vi "N5700 Reset.vi"(5 "error":errorcluster, 8 "VISA":refnum<visa-resource-name>) -> (0 "error out":errorcluster, 3 "VISA out":refnum<visa-resource-name>)   [LabVIEW 2020]
doc: "This VI resets the N5700 power supply to a precise and safe state. \n\nThe reset state includes:\n- Output off\n- Voltage program limit to zero\n- Current program limit to zero\n- Over-voltage protection setting to maximum\n- Under-voltage limit to zero\n- Over-current protection off\n\nStatus registers are not reset"
panel:
  in  "Command":string="*RST"
  # "Agilent Technologies  \nSeries N5700A\n  DC Power Supplies"
  # "Reset Power Supply"
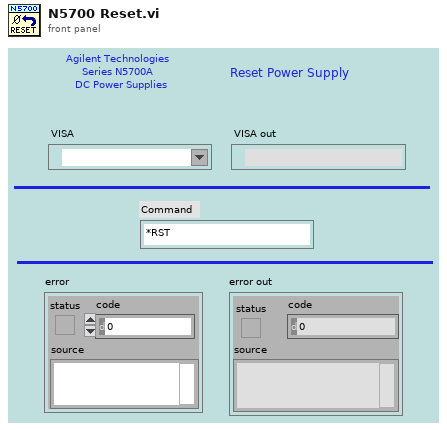
[diagram p1: front panel]
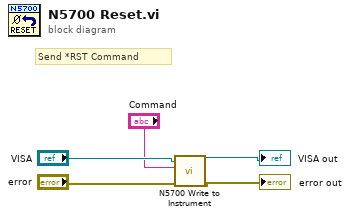
[diagram p0: block diagram]
diagram:
  # "Send *RST Command"
  n1 = call "N5700 Write to Instrument.vi"("error"="error", "Command"="Command", "VISA"="VISA") -> ("error out"=→"error out":errorcluster, "VISA out"=→"VISA out":refnum<visa-resource-name>)  [unwired: 4 in]
